vi "Get Q Factor.vi"(5 "X":dbl[](array[numeric]), 6 "Y":dbl[](array[numeric]), 7 "Error In":errorcluster) -> (0 "Fitted Data":waveform(dbl), 1 "best fit parameters":dbl[](array[numeric]), 2 "Q Factor":dbl, 3 "error out":errorcluster, 4 "covariance":T1)   [LabVIEW 2015, in "Math Utilities.lvlib"]
doc: "<B>Get Q Factor</B> fits the resonant a frequency domain signal returned from an FFT over a predefined frequency range using a Lorentzian, non-parametric curve fitting model. This VI returns the best fit parameters, the third factor being the resonant frequency of the fit, the fitted data and te Q factor.\n\nThe Q factor defines the quality of the resonator. According to Miklos et al. (2001, Rev. Sci. Instr.), this factor is defined as the product of twice Pi and the accumulated energy over the energy lost over one period, or the fundamental frequency over the half-width of the resonant profile.\n\nCHANGED 2/7/2012 to reflect correct Q calculation."
uses:
  Math Utilities.lvlib
  <vilib>/Analysis/Matrix/Datatypes/RealMatrix.ctl
  <vilib>/gmath/NumericalOptimization/Nonlinear Curve Fit LM.vi
  <vilib>/gmath/NI_Gmath.lvlib
  <vilib>/Analysis/Matrix/NI_Matrix.lvlib
panel:
  out "number of function calls":i32
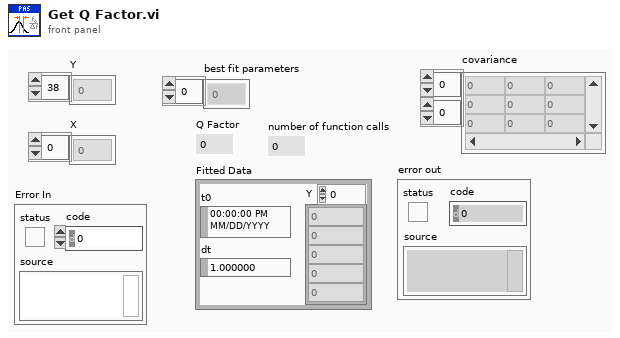
[diagram p1: front panel]
types:
  T1 = typedef "NI_Matrix.lvlib/RealMatrix.ctl" = dbl[][]
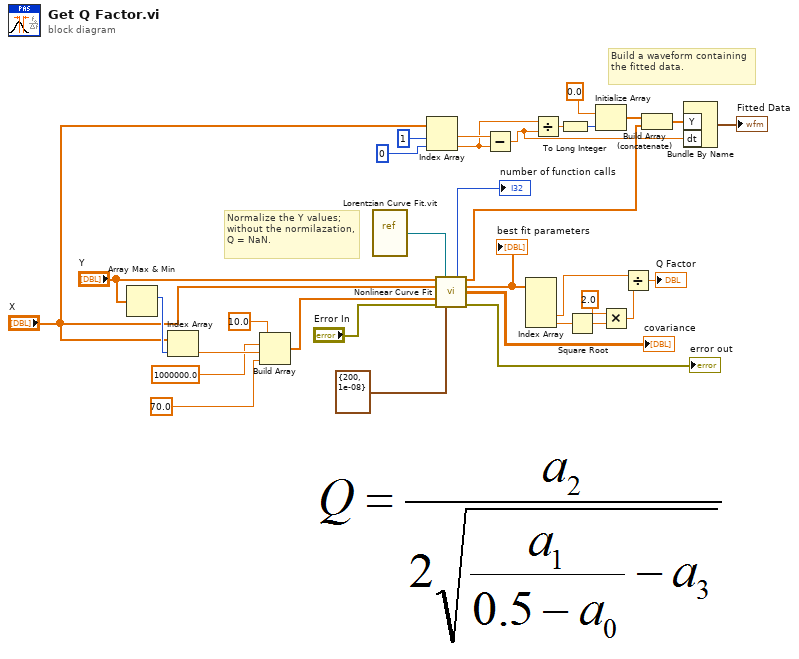
[diagram p0: block diagram]
diagram:
  # "Build a waveform containing the fitted data."
  # "Normalize the Y values; without the normilazation, Q = NaN."
  n1 = Array Max & Min(array="Y") -> (max index (indices)=w32:i32)  [unwired: 3 out]
  n2 = Index Array(array="X", index=w32) -> (element=w31:dbl)
  n3 = Build Array(10.0 ("element"), 1000000.0 ("element"), w31, 70.0 ("element")) -> (w30:dbl[])
  n4 = vi-ref "Lorentzian Curve Fit.vit"() -> (w33:refnum<vi>)
  n5 = Index Array(array="X", index #1=1 ("index"), index #2=0 ("index")) -> (element #1=w25:dbl, element #2=w24:dbl)
  n6 = call-poly <vilib>:"Nonlinear Curve Fit.vi"("Y"="Y", "f(x,a)"=w33, "X"="X", "initial parameters"=w30, "error in (no error)"="Error In", "termination"=cluster{"max iteration":i32, "tolerance":dbl} {"max iteration"=200, "tolerance"=1e-08}) -> ("number of function calls"=→"number of function calls":i32, "best nonlinear fit"=w17:dbl[], "best fit parameters"=w15:dbl[], "covariance"=→"covariance":T1, "error out"=→"error out":errorcluster)  [unwired: 2 in, 3 out]
  "best fit parameters" <- w15
  n7 = Subtract(x=w25, y=w24) -> (x-y=w3:dbl)
  n8 = Index Array(array=w15) -> (element #3=w14:dbl, element #4=w13:dbl)  [unwired: 4 in, 2 out]
  n9 = Divide(x=w24, y=w3) -> (x/y=w5:dbl)
  n10 = To Long Integer(number=w5) -> (32bit integer=w4:i32)
  n11 = Square Root(x=w13) -> (sqrt(x)=w12:dbl)
  n12 = Initialize Array(0.0 ("element"), w4) -> (w22:dbl[])
  n13 = Multiply(x=2.0, y=w12) -> (x*y=w10:dbl)
  n14 = Divide(x=w14, y=w10) -> (x/y=→"Q Factor":dbl)
  n15 = Build Array (concatenate)(w22, w17) -> (w2:dbl[])
  n16 = Bundle By Name("Y"=w2, "dt"=w3) -> (→"Fitted Data":waveform(dbl))  [unwired: 1 out]
